vi "get_lib_path.vi"() -> (0 "Path":path)   [LabVIEW 2015]
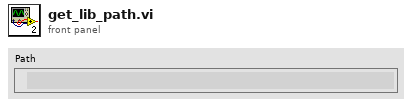
[diagram p1: front panel]
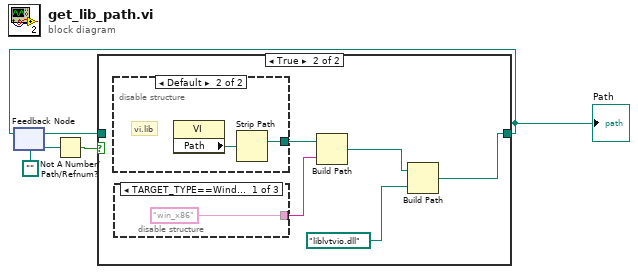
[diagram p0: block diagram]
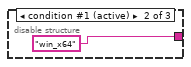
[diagram p3: hidden frame]
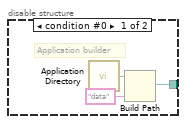
[diagram p5: hidden frame]
diagram:
  n1 = feedback #1(path "") -> (w2:path)
  n2 = Not A Number/Path/Refnum?(number/path/refnum=w2) -> (NaN/Path/Refnum?=w3:bool)
  n3 = case shown="True" w3 {
    tunnel: w2 -> [w5 _]
    tunnel: [w5 w7] -> w1
    frame False {
    }
    frame True {
      n4 = disable-structure shown="Default" {
        disable-tunnel: [w15 w17] -> w10
        frame condition #0 {
          # "Application builder"
          n5 = call <vilib>:"Application Directory.vi"() -> ("Application Directory"=w13:path)
          n6 = Build Path(base path=w13, name or relative path="data") -> (appended path=w15:path)
        }
        frame condition #1 (active) {
          # "vi.lib"
          n7 = property class="VI"() -> ("Path"=w16:path)  [unwired: 2 in, 2 out]
          n8 = Strip Path(path=w16) -> (stripped path=w17:path)  [unwired: 1 out]
        }
      }
      n9 = disable-structure shown="TARGET_TYPE==Windows&&TARGET_BITNESS==32" {
        disable-tunnel: ["win_x86" ("name") "win_x64" ("name") _] -> w9
        frame condition #0 {
        }
        frame condition #1 (active) {
        }
        frame condition #2 {
        }
      }
      n10 = Build Path(base path=w10, name or relative path=w9) -> (appended path=w8:path)
      n11 = Build Path(base path=w8, name or relative path=path "liblvtvio.dll" ("appended path")) -> (appended path=w7:path)
    }
  }
  "Path" <- w1
  n12 = feedback-in #1(w1) -> ()
